vi "AWG Waveform Generator_Edited.vi"() -> ()   [LabVIEW 2020]
doc: "This example shows how to use the Arbitrary Waveform mode."
uses:
  <instrlib>/niFgen/niFgen.llb/niFgen Output Mode.ctl
  <instrlib>/niFgen/niFgen.llb/niFgen Trigger Mode.ctl
  <instrlib>/niFgen/niFgen.llb/niFgen Create Waveform (WDT).vi
panel:
  out "NaN/Path/Refnum?":bool
  out "Waveform Graph 2":waveform(dbl)(graph)
  in  "Transient":T1={"t1 (ms)"=10.0, "t2 (ms)"=10.0, "t3 (ms)"=10.0, "High Load (A)"=1.0, "Low Load (A)"=0.0, "Slew rate A/us"=0.001}
  in  "error out":errorcluster
  out "Max Waveform size-Read":i32 format="%_1p"
  out "Waveform Graph":waveform(dbl)(graph)
  in  "Update":bool
  in  "Stop":bool
  in  "FGEN Resource Name":refnum<k15>
  out "Actual Sample Rate (S/s)":dbl format="%.2p"
  in  "Sample Rate (S/s)":dbl=20000000.0 format="%.2p"
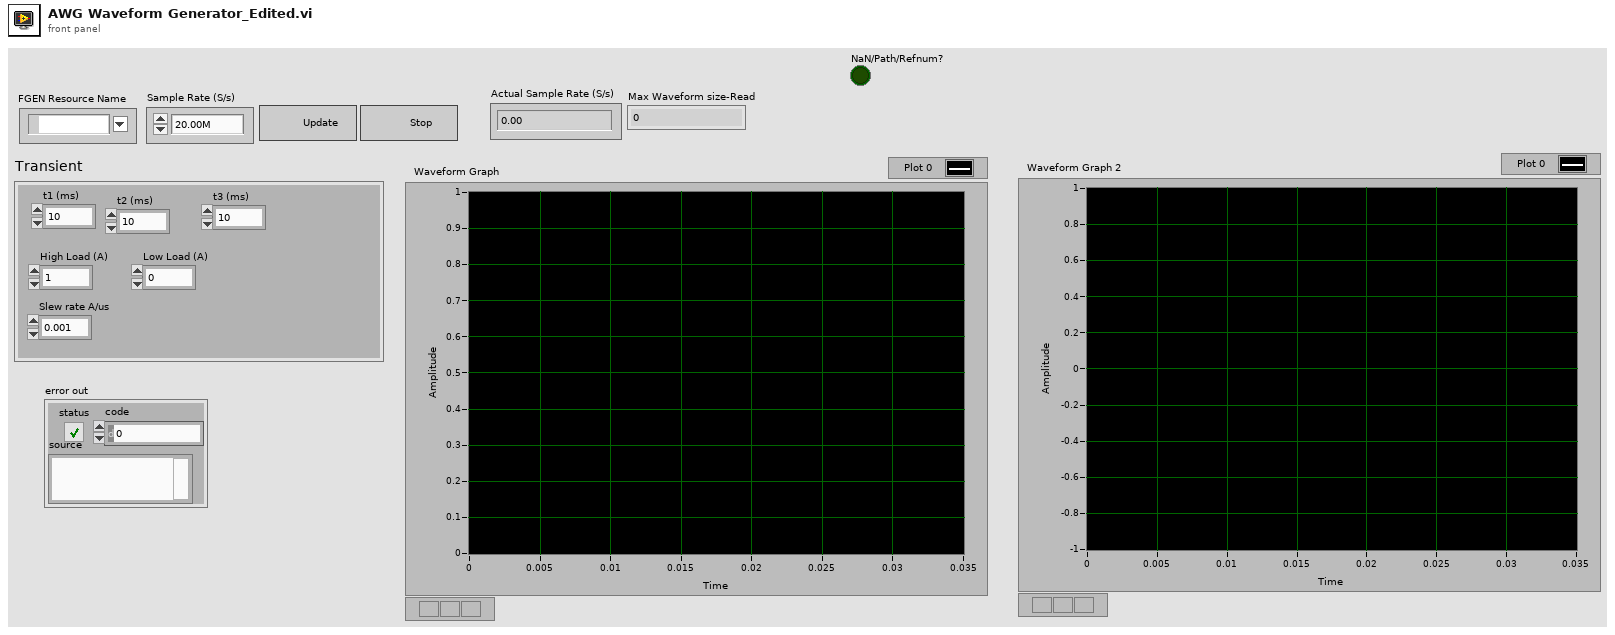
[diagram p1: front panel]
types:
  T1 = cluster{"t1 (ms)":dbl, "t2 (ms)":dbl, "t3 (ms)":dbl, "High Load (A)":dbl, "Low Load (A)":dbl, "Slew rate A/us":dbl}
  T2 = typedef "niFgen Trigger Mode.ctl" = i32
  T3 = typedef "niFgen Output Mode.ctl" = u32
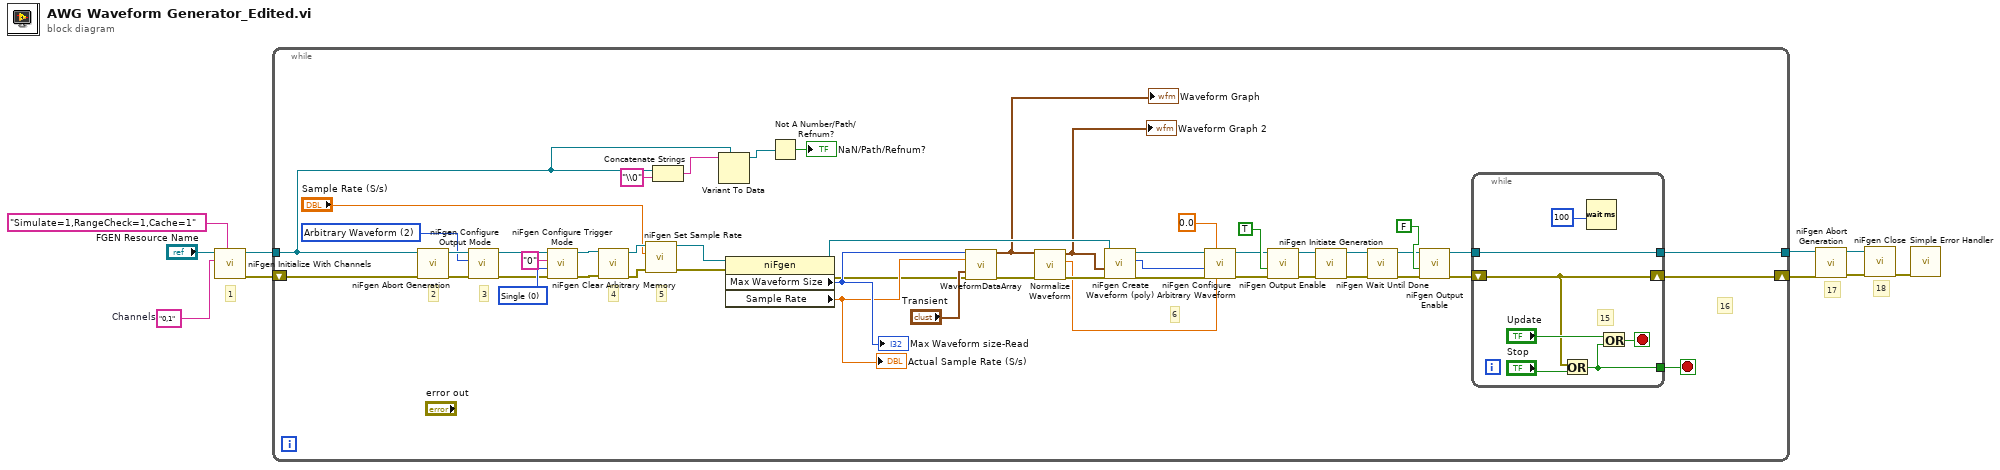
[diagram p0: block diagram]
diagram:
  w4 = "0,1"  # Channels
  # "18"
  # "17"
  # "1"
  n1 = call <instrlib>:"niFgen Initialize With Channels.vi"("Option String"="Simulate=1,RangeCheck=1,Cache=1", "Channel Name"=w4, "Resource Name"="FGEN Resource Name") -> ("error out"=w3:errorcluster, "Instrument Handle Out"=w1:refnum<k15>)  [unwired: 7 in]
  n2 = while {
    tunnel: [w22] -> w10
    tunnel: w1 -> [w13]
    shift-right: [w24] -> w6
    shift-left: w3 -> [w50]
    stop <- w49 stop-if-true
    w39 = T2 0 items=["Single", "Continuous", "Stepped", "Burst"] ("Trigger Mode")
    w52 = T3 2 items=["Standard Function", "Frequency List", "Arbitrary Waveform", "Arbitrary Sequence", "Script"] ("Output Mode")
    # "16"
    # "6"
    # "5"
    # "4"
    # "3"
    # "2"
    n3 = call <instrlib>:"niFgen Abort Generation.vi"("error in (no error)"=w50, "Instrument Handle"=w13) -> ("error out"=w56:errorcluster, "Instrument Handle Out"=w55:refnum<k15>)  [unwired: 8 in]
    n4 = call <instrlib>:"niFgen Configure Output Mode.vi"("error in (no error)"=w56, "Output Mode (default: 0=Standard Function)"=w52, "Instrument Handle"=w55) -> ("error out"=w37:errorcluster, "Instrument Handle Out"=w38:refnum<k15>)  [unwired: 6 in]
    n5 = call <instrlib>:"niFgen Configure Trigger Mode.vi"("error in (no error)"=w37, "Trigger Mode (default: 1=continuous)"=w39, "Channel Name"="0", "Instrument Handle"=w38) -> ("error out"=w35:errorcluster, "Instrument Handle Out"=w36:refnum<k15>)  [unwired: 6 in]
    n6 = call <instrlib>:"niFgen Clear Arbitrary Memory.vi"("error in (no error)"=w35, "Instrument Handle"=w36) -> ("error out"=w45:errorcluster, "Instrument Handle Out"=w46:refnum<k15>)  [unwired: 8 in]
    n7 = call <instrlib>:"niFgen Set Sample Rate.vi"("error in (no error)"=w45, "Sample Rate (Samp/s)"="Sample Rate (S/s)", "Instrument Handle"=w46) -> ("error out"=w40:errorcluster, "Instrument Handle Out"=w41:refnum<k15>)  [unwired: 7 in]
    n8 = Concatenate Strings(w13, "\\0" ("string")) -> (w14:string)
    n9 = Variant To Data(type=w13, Variant=w14) -> (data=w12:refnum<k15>)  [unwired: 1 in, 1 out]
    n10 = property class="niFgen"(reference=w41, error in=w40) -> (reference out=w29:refnum<k15>, error out=w31:errorcluster, "Max Waveform Size"=w33:i32, "Sample Rate"=w32:dbl)
    "Actual Sample Rate (S/s)" <- w32
    "Max Waveform size-Read" <- w33
    n11 = Not A Number/Path/Refnum?(number/path/refnum=w12) -> (NaN/Path/Refnum?=→"NaN/Path/Refnum?":bool)
    n12 = call "WaveformDataArray.vi"("Max Waveform Size"=w33, "Sample Rate"=w32, "Transient"="Transient", "error in"=w31) -> ("Waveform Graph 2"=w19:waveform(dbl), "error out"=w30:errorcluster)  [unwired: 9 in, 1 out]
    "Waveform Graph" <- w19
    n13 = call <vilib>:"Normalize Waveform.vi"("error in (no error)"=w30, "waveform in"=w19) -> ("error out"=w21:errorcluster, "scale"=w20:dbl, "normalized waveform"=w18:waveform(dbl))  [unwired: 6 in, 1 out]
    "Waveform Graph 2" <- w18
    n14 = call-poly <instrlib>:"niFgen Create Waveform (poly).vi"("error in (no error)"=w21, "Waveform"=w18, "Instrument Handle"=w29) -> ("error out"=w57:errorcluster, "Waveform Handle"=w47:i32, "Instrument Handle Out"=w58:refnum<k15>)  [unwired: 6 in]
    n15 = call <instrlib>:"niFgen Configure Arbitrary Waveform.vi"("Gain"=w20, "Offset"=0.0, "error in (no error)"=w57, "Waveform Handle"=w47, "Instrument Handle"=w58) -> ("error out"=w42:errorcluster, "Instrument Handle Out"=w43:refnum<k15>)  [unwired: 5 in]
    n16 = call <instrlib>:"niFgen Output Enable.vi"("error in (no error)"=w42, "Output Enable (default: True)"=TRUE ("output enable"), "Instrument Handle"=w43) -> ("error out"=w53:errorcluster, "Instrument Handle Out"=w54:refnum<k15>)  [unwired: 7 in]
    n17 = call <instrlib>:"niFgen Initiate Generation.vi"("error in (no error)"=w53, "Instrument Handle"=w54) -> ("error out"=w27:errorcluster, "Instrument Handle Out"=w28:refnum<k15>)  [unwired: 8 in]
    n18 = call <instrlib>:"niFgen Wait Until Done.vi"("error in (no error)"=w27, "Instrument Handle"=w28) -> ("error out"=w25:errorcluster, "Instrument Handle Out"=w26:refnum<k15>)  [unwired: 8 in]
    n19 = call <instrlib>:"niFgen Output Enable.vi"("error in (no error)"=w25, "Output Enable (default: True)"=FALSE ("output enable"), "Instrument Handle"=w26) -> ("error out"=w24:errorcluster, "Instrument Handle Out"=w23:refnum<k15>)  [unwired: 7 in]
    n20 = while {
      tunnel: w23 -> [w60]
      tunnel: [w61] -> w49
      tunnel: [w60] -> w22
      shift-right: [w59] -> _
      shift-left: w24 -> [w59]
      stop <- w64 stop-if-true
      # "The case structure ensures that only valid values \nare used for DC Offset because the offset values \ndependent on the configured Gain Value."
      # "15"
      n21 = Or(x=w59, y="Stop") -> (x .or. y?=w61:bool)
      n22 = Wait (ms)(milliseconds to wait=u32 100 ("millisecond multiple")) -> ()  [unwired: 1 out]
      n23 = Or(x="Update", y=w61) -> (x .or. y?=w64:bool)
    }
  }
  n24 = call <instrlib>:"niFgen Abort Generation.vi"("error in (no error)"=w6, "Instrument Handle"=w10) -> ("error out"=w9:errorcluster, "Instrument Handle Out"=w8:refnum<k15>)  [unwired: 8 in]
  n25 = call <instrlib>:"niFgen Close.vi"("error in (no error)"=w9, "Instrument Handle"=w8) -> ("error out"=w7:errorcluster)  [unwired: 9 in]
  n26 = call <vilib>:"Simple Error Handler.vi"("error in (no error)"=w7) -> ()  [unwired: 4 in, 5 out]
